vi "Get RGA Numerical Parameter.vi"(3 "error in (no error)":errorcluster, 4 "Command":string, 5 "Port Number":refnum<visa-resource-name>) -> (0 "error out":errorcluster, 1 "Parameter":dbl format="%.2f")   [LabVIEW 2019]
uses:
  Serial Support VISA.llb/Serial Actions.ctl
panel:
  out "Serial Read":string
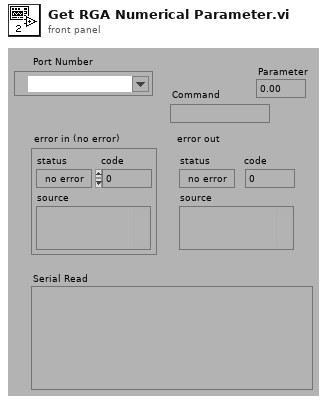
[diagram p1: front panel]
types:
  T1 = typedef "Serial Actions.ctl" = enum16{"Init", "Break", "Clear Buffer", "Write", "Read", "N Bytes", "Lock", "Unlock", "Close"}
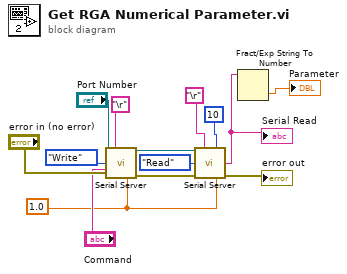
[diagram p0: block diagram]
diagram:
  w8 = 1.0
  n1 = call "Serial Server.vi"("VISA Resource Name"="Port Number", "EOT Chars (cr/lf)"="\r", "Action"=Serial_Actions."Write", "String To Send"="Command", "error in (no error)"="error in (no error)", "Timeout Limit(sec)"=w8) -> ("dup VISA Resource Name"=w2:refnum<visa-resource-name>, "error out"=w3:errorcluster)  [unwired: 5 in, 3 out]
  n2 = call "Serial Server.vi"("VISA Resource Name"=w2, "EOT Chars (cr/lf)"="\r", "Max Char to Read"=10, "Action"=Serial_Actions."Read", "error in (no error)"=w3, "Timeout Limit(sec)"=w8) -> ("Serial Read"=w5:string, "error out"=→"error out":errorcluster)  [unwired: 5 in, 3 out]
  "Serial Read" <- w5
  n3 = Fract/Exp String To Number(string=w5) -> (number=→"Parameter":dbl)  [unwired: 3 in, 1 out]
